vi "SonarSweep.vi"() -> ()   [LabVIEW 2014]
uses:
  <vilib>/Instr/_visa.llb/VISA Flush IO Buffer Mask.ctl
  <vilib>/Instr/_visa.llb/VISA Configure Serial Port (Instr).vi
  <vilib>/Utility/file.llb/Write To Spreadsheet File (DBL).vi
panel:
  out "Position":i32
  in  "file path":path
  out "Waveform Chart":dbl(graph)
  out "Distance, in":dbl
  in  "stop":bool
  out "error out":errorcluster
  out "return count":u32
  out "read buffer":string
  in  "VISA resource name":refnum<visa-resource-name>="COM3"
  # "This vi reads a continuous stream of data from the Senix Sonix sensor TSPC-30S1-232\nThe sensor has been configured to stream continuous data using their software SenixView.\nThe serial port setup values are the default for the Senix sensor."
  # "The value 0000 represent \"no read\""
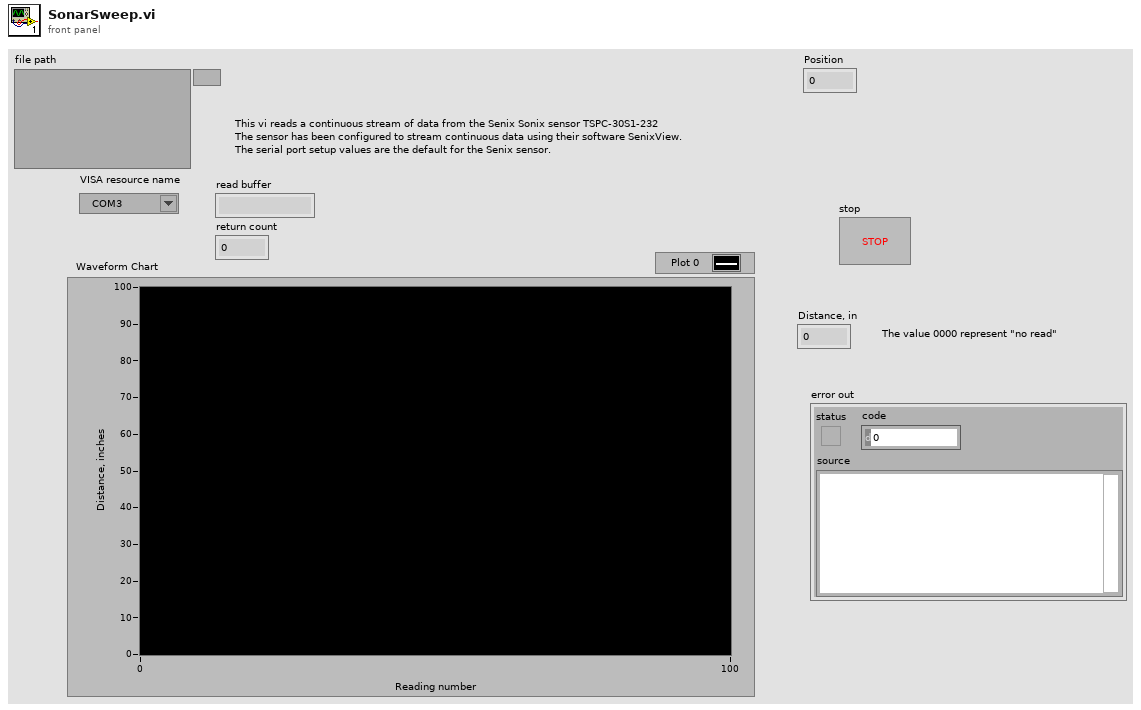
[diagram p1: front panel]
types:
  T1 = typedef "VISA Flush IO Buffer Mask.ctl" = u16
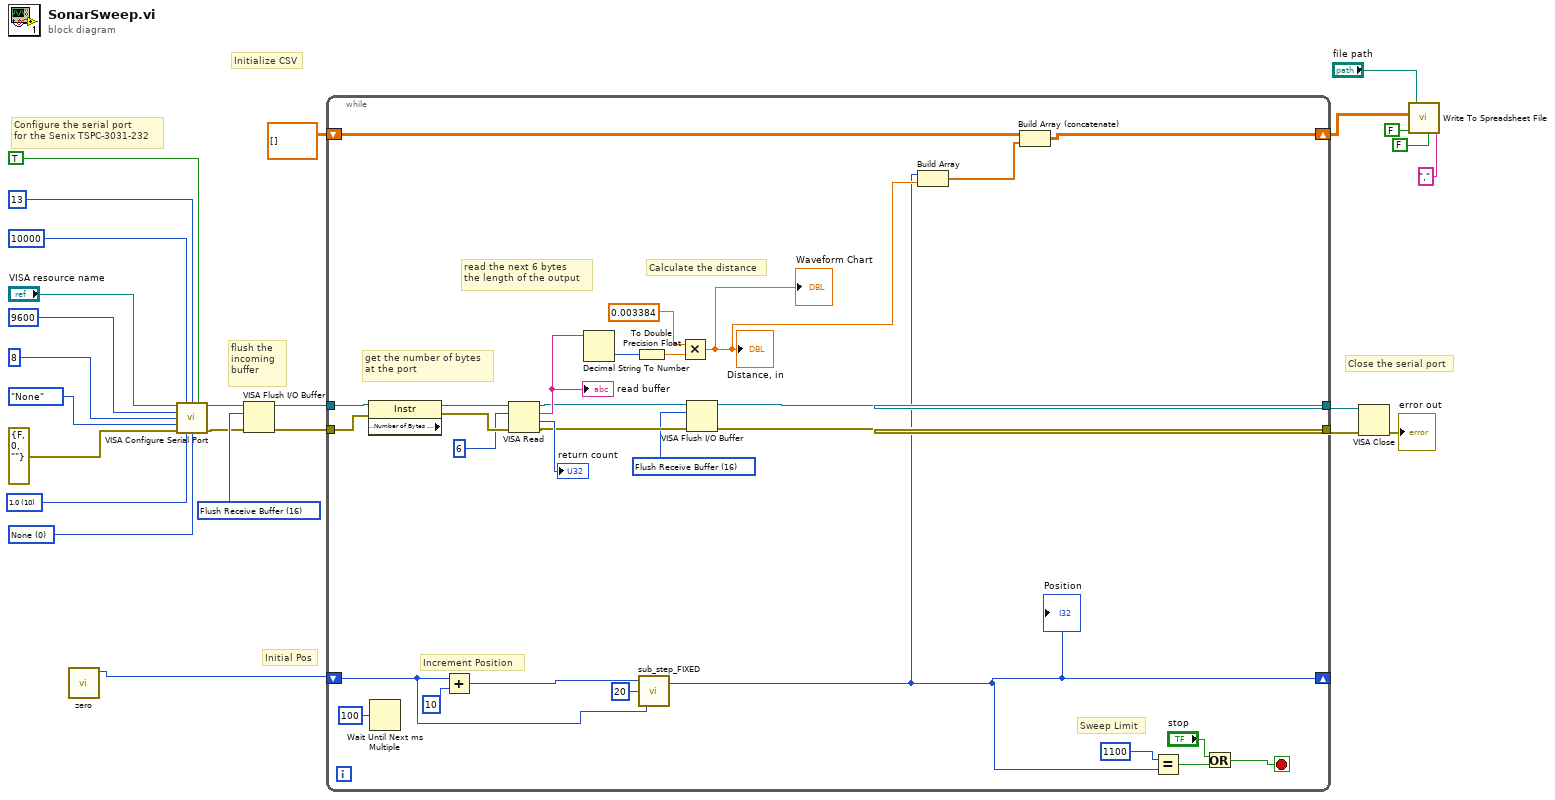
[diagram p0: block diagram]
diagram:
  w12 = T1 16 items=["Flush Receive Buffer"=16, "Write Transmit Buffer to Device"=32, "Flush Receive Buffer (No I/O)"=64, "Flush Transmit Buffer"=128] ("Mask")
  w19 = u16 0 items=["None", "XON/XOFF", "RTS/CTS", "XON/XOFF & RTS/CTS", "DTR/DSR", "XON/XOFF & DTR/DSR"] ("flow control (0:none)")
  w21 = u16 10 items=["1.0"=10, "1.5"=15, "2.0"=20] ("stop bits (10: 1 bit)")
  # "Initialize CSV"
  # "Initial Pos"
  # "Close the serial port"
  # "flush the \nincoming \nbuffer"
  # "Configure the serial port\nfor the Senix TSPC-3031-232"
  n1 = call "zero.vi"() -> ("PositionOut"=w1:i32)  [unwired: 11 in]
  n2 = call-poly "VISA Configure Serial Port"("VISA resource name"="VISA resource name", "timeout (10sec)"=u32 10000, "termination char\n(0xA = '\\n' = LF)"=u8 13 ("termination char\n(0xA = '\\n' = LF)"), "Enable Termination\nChar (T)"=TRUE ("Enable Termination\nChar (T)"), "baud rate (9600)"=u32 9600, "data bits (8)"=u16 8, "parity (0:none)"=enum16{"None", "Odd", "Even", "Mark", "Space"}."None", "error in (no error)"=errorcluster {"status"=FALSE, "code"=0, "source"=""}, "stop bits (10: 1 bit)"=w21, "flow control (0:none)"=w19) -> ("VISA resource name out"=w11:refnum<visa-resource-name>, "error out"=w10:errorcluster)  [unwired: 4 in]
  n3 = VISA Flush I/O Buffer(VISA resource name=w11, mask (16)=w12, error in (no error)=w10) -> (VISA resource name out=w9:refnum<visa-resource-name>, error out=w8:errorcluster)
  n4 = while {
    tunnel: [w44] -> w15
    tunnel: [w43] -> w14
    tunnel: w9 -> [w49]
    tunnel: w8 -> [w48]
    shift-right: [w27] -> _
    shift-left: w1 -> [w28]
    shift-right: [w32] -> w6
    shift-left: dbl[][] [] -> [w33]
    stop <- w35 stop-if-true
    w40 = T1 16 items=["Flush Receive Buffer"=16, "Write Transmit Buffer to Device"=32, "Flush Receive Buffer (No I/O)"=64, "Flush Transmit Buffer"=128] ("Mask")
    # "Sweep Limit"
    # "Increment Position"
    # "Calculate the distance"
    # "read the next 6 bytes\nthe length of the output"
    # "get the number of bytes\nat the port"
    n5 = property class="Instr" props=["Serial Settings:Number of Bytes at Serial Port"](reference=w49, error in=w48) -> (reference out=w54:refnum<visa-resource-name>, error out=w53:errorcluster)  [unwired: 1 out]
    n6 = Wait Until Next ms Multiple(millisecond multiple=u32 100) -> ()  [unwired: 1 out]
    n7 = Add(x=w28, y=10) -> (x+y=w29:i32)
    n8 = VISA Read(VISA resource name=w54, byte count=u32 6, error in (no error)=w53) -> (VISA resource name out=w42:refnum<visa-resource-name>, read buffer=w51:string, return count=→"return count":u32, error out=w41:errorcluster)
    "read buffer" <- w51
    n9 = Decimal String To Number(string=w51) -> (number=w47:i32)  [unwired: 2 in, 1 out]
    n10 = To Double Precision Float(number=w47) -> (double precision float=w46:dbl)
    n11 = call "sub_step_FIXED.vi"("Current Position"=w28, "millisecond multiple"=u32 20, "Desired Position"=w29) -> ("Position Out"=w27:i32)  [unwired: 1 in]
    "Position" <- w27
    n12 = Multiply(x=0.003384, y=w46) -> (x*y=w30:dbl)
    "Distance, in" <- w30
    "Waveform Chart" <- w30
    n13 = VISA Flush I/O Buffer(VISA resource name=w42, mask (16)=w40, error in (no error)=w41) -> (VISA resource name out=w44:refnum<visa-resource-name>, error out=w43:errorcluster)
    n14 = Build Array(w27, w30) -> (w31:dbl[])
    n15 = Build Array (concatenate)(w33, w31) -> (w32:dbl[][])
    n16 = Equal?(x=1100 ("y"), y=w27) -> (x = y?=w37:bool)
    n17 = Or(x="stop", y=w37) -> (x .or. y?=w35:bool)
  }
  n18 = VISA Close(VISA resource name=w15, error in (no error)=w14) -> (error out=→"error out":errorcluster)
  n19 = call-poly <vilib>:"Write To Spreadsheet File.vi"("delimiter (\\t)"="," ("delimiter (\\t)"), "transpose? (no:F)"=FALSE, "append to file? (new file:F)"=FALSE, "2D data"=w6, "file path (dialog if empty)"="file path") -> ()  [unwired: 3 in, 1 out]
